vi "ADD ITEM TO CHECKOUT.vi"(10 "REFERENCES":T2, 11 "DATA IN":T1[](array[typedef])) -> (3 "DATA OUT":T1[](array[typedef]))   [LabVIEW 2019]
uses:
  Controls/References Cluster.ctl
  Controls/Custom Calendar/Custom Calendar.xctl
  Controls/Table Data Types/Inventory Data Type.ctl
  <vilib>/addons/database/Connection.llb/DB Tools Open Connec (String).vi
  <vilib>/addons/database/_DB Variant To Data/Database Variant To Data.xnode
  <vilib>/addons/database/NI_Database_API.lvlib
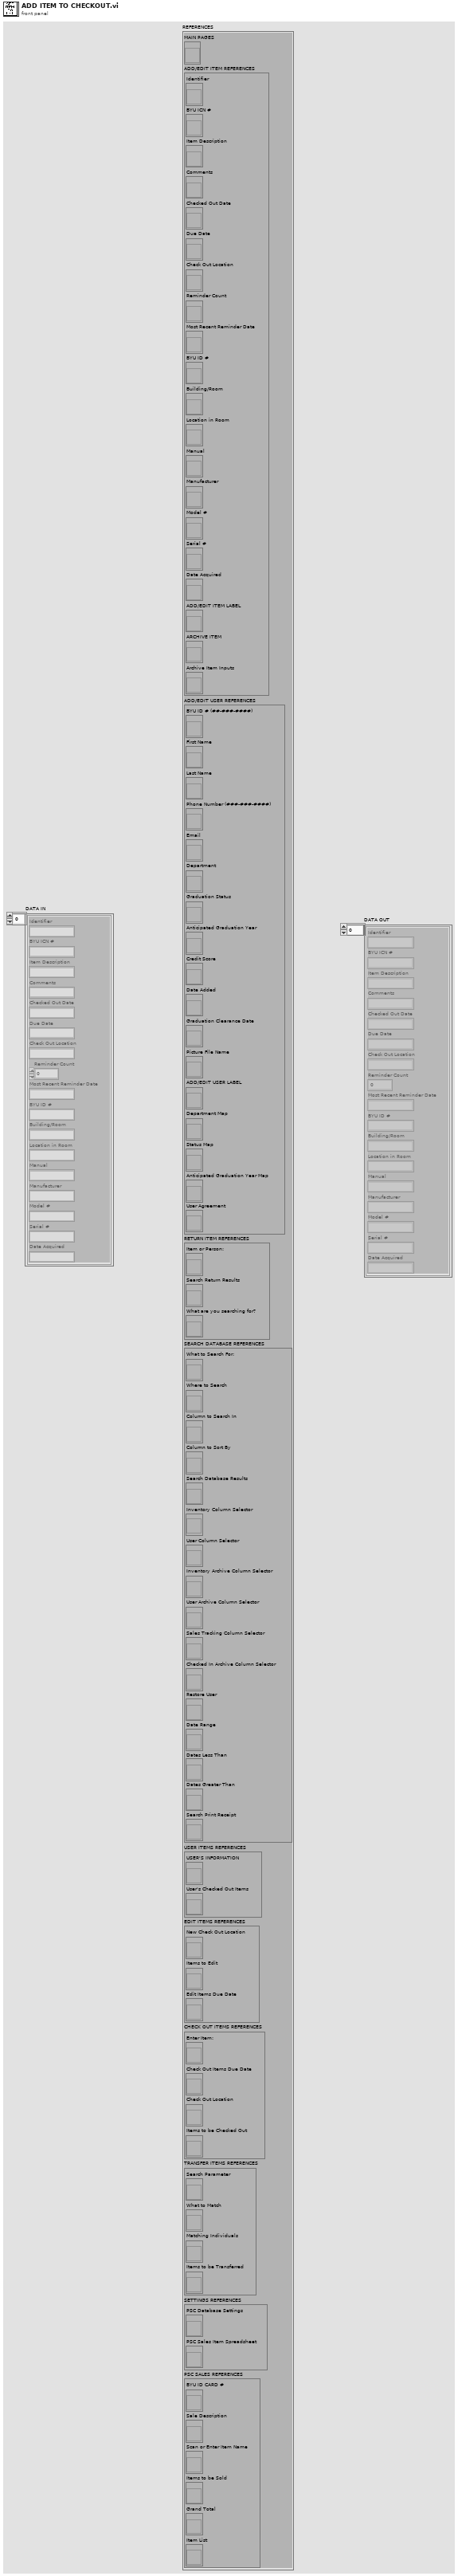
[diagram p1: front panel]
types:
  T1 = typedef "Inventory Data Type.ctl" = cluster{"Identifier":string, "BYU ICN #":string, "Item Description":string, "Comments":string, "Checked Out Date":string, "Due Date":string, "Check Out Location":string, "Reminder Count":i32, "Most Recent Reminder Date":string, "BYU ID #":string, "Building/Room":string, "Location in Room":string, "Manual":string, "Manufacturer":string, "Model #":string, "Serial #":string, "Date Acquired":string}
  T2 = typedef "References Cluster.ctl" = cluster{"MAIN PAGES":refnum<vi>, "ADD/EDIT ITEM REFERENCES":cluster{"Identifier":refnum<vi>, "BYU ICN #":refnum<vi>, "Item Description":refnum<vi>, "Comments":refnum<vi>, "Checked Out Date":refnum<vi>, "Due Date":refnum<vi>, "Check Out Location":refnum<vi>, "Reminder Count":refnum<vi>, "Most Recent Reminder Date":refnum<vi>, "BYU ID #":refnum<vi>, "Building/Room":refnum<vi>, "Location in Room":refnum<vi>, "Manual":refnum<vi>, "Manufacturer":refnum<vi>, "Model #":refnum<vi>, "Serial #":refnum<vi>, "Date Acquired":refnum<vi>, "ADD/EDIT ITEM LABEL":refnum<vi>, "ARCHIVE ITEM":refnum<vi>, "Archive Item Inputs":refnum<vi>}, "ADD/EDIT USER REFERENCES":cluster{"BYU ID # (##-###-####)":refnum<vi>, "First Name":refnum<vi>, "Last Name":refnum<vi>, "Phone Number (###-###-####)":refnum<vi>, "Email":refnum<vi>, "Department":refnum<vi>, "Graduation Status":refnum<vi>, "Anticipated Graduation Year":refnum<vi>, "Credit Score":refnum<vi>, "Date Added":refnum<vi>, "Graduation Clearance Date":refnum<vi>, "Picture File Name":refnum<vi>, "ADD/EDIT USER LABEL":refnum<vi>, "Department Map":refnum<vi>, "Status Map":refnum<vi>, "Anticipated Graduation Year Map":refnum<vi>, "User Agreement":refnum<vi>}, "RETURN ITEM REFERENCES":cluster{"Item or Person:":refnum<vi>, "Search Return Results":refnum<vi>, "What are you searching for?":refnum<vi>}, "SEARCH DATABASE REFERENCES":cluster{"What to Search For:":refnum<vi>, "Where to Search":refnum<vi>, "Column to Search In":refnum<vi>, "Column to Sort By":refnum<vi>, "Search Database Results":refnum<vi>, "Inventory Column Selector":refnum<vi>, "User Column Selector":refnum<vi>, "Inventory Archive Column Selector":refnum<vi>, "User Archive Column Selector":refnum<vi>, "Sales Tracking Column Selector":refnum<vi>, "Checked In Archive Column Selector":refnum<vi>, "Restore User":refnum<vi>, "Date Range":refnum<vi>, "Dates Less Than":refnum<vi>, "Dates Greater Than":refnum<vi>, "Search Print Receipt":refnum<vi>}, "USER ITEMS REFERENCES":cluster{"USER'S INFORMATION":refnum<vi>, "User's Checked Out Items":refnum<vi>}, "EDIT ITEMS REFERENCES":cluster{"New Check Out Location":refnum<vi>, "Items to Edit":refnum<vi>, "Edit Items Due Date":refnum<vi>}, "CHECK OUT ITEMS REFERENCES":cluster{"Enter Item:":refnum<vi>, "Check Out Items Due Date":refnum<vi>, "Check Out Location":refnum<vi>, "Items to be Checked Out":refnum<vi>}, "TRANSFER ITEMS REFERENCES":cluster{"Search Parameter":refnum<vi>, "What to Match":refnum<vi>, "Matching Individuals":refnum<vi>, "Items to be Transferred":refnum<vi>}, "SETTINGS REFERENCES":cluster{"PSC Database Settings":refnum<vi>, "PSC Sales Item Spreadsheet":refnum<vi>}, "PSC SALES REFERENCES":cluster{"BYU ID CARD #":refnum<vi>, "Sale Description":refnum<vi>, "Scan or Enter Item Name":refnum<vi>, "Items to be Sold":refnum<vi>, "Grand Total":refnum<vi>, "Item List":refnum<vi>}}
  T3 = cluster{"Enter Item:":refnum<vi>, "Check Out Items Due Date":refnum<vi>, "Check Out Location":refnum<vi>, "Items to be Checked Out":refnum<vi>}
  T4 = typedef "NI_Database_API.lvlib/Conn ObjectReference.ctl" = refnum<k1>
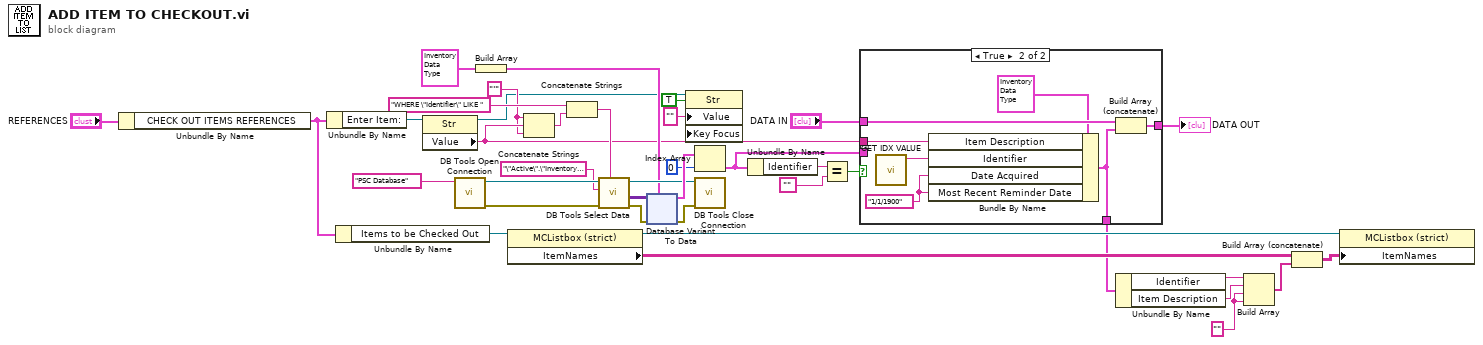
[diagram p0: block diagram]
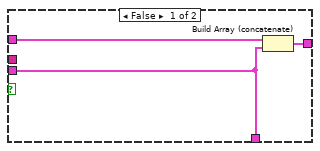
[diagram p2: hidden frame]
diagram:
  w4 = "" ("element")
  w16 = "'"
  n1 = Unbundle By Name("REFERENCES") -> ("CHECK OUT ITEMS REFERENCES"=w14:T3)
  n2 = Unbundle By Name(w14) -> ("Enter Item:"=w37:refnum<vi>)
  n3 = Unbundle By Name(w14) -> ("Items to be Checked Out"=w13:refnum<vi>)
  n4 = property class="Str"(reference=w37) -> (reference out=w3:refnum<vi>, "Value"=w17:string)  [unwired: 1 in, 1 out]
  n5 = call-poly <vilib>:"DB Tools Open Connection.vi"("connection information"="PSC Database") -> ("error out"=w35:errorcluster, "connection reference"=w36:T4)  [unwired: 7 in]
  n6 = Build Array(T1 {"Identifier"="", "BYU ICN #"="", "Item Description"="", "Comments"="", "Checked Out Date"="", "Due Date"="", "Check Out Location"="", "Reminder Count"=0, "Most Recent Reminder Date"="", "BYU ID #"="", "Building/Room"="", "Location in Room"="", "Manual"="", "Manufacturer"="", "Model #"="", "Serial #"="", "Date Acquired"=""} ("Array")) -> (w19:T1[])
  n7 = property class="MCListbox (strict)"(reference=w13) -> (reference out=w8:refnum<vi>, "ItemNames"=w10:string[][])  [unwired: 1 in, 1 out]
  n8 = Concatenate Strings(w16, w17, w16) -> (w18:string)
  n9 = Concatenate Strings("WHERE \"Identifier\" LIKE ", w18) -> (w32:string)
  n10 = call <vilib>:"DB Tools Select Data.vi"("condition"=w32, "error in (no error)"=w35, "table"="\"Active\".\"Inventory\"", "connection reference"=w36) -> ("error out"=w30:errorcluster, "data"=w31:variant[][], "connection reference out"=w27:T4)  [unwired: 2 in]
  n11 = xnode "Database Variant To Data"("database variant"=w31, "error in (no error)"=w30, "type"=w19) -> ("data"=w29:T1[], "error out"=w26:errorcluster)
  n12 = property class="Str"(reference=w3, "Value"="", "Key Focus"=TRUE) -> ()  [unwired: 1 in, 2 out]
  n13 = Index Array(array=w29, index=0) -> (element=w15:T1)
  n14 = call <vilib>:"DB Tools Close Connection.vi"("error in (no error)"=w26, "connection reference"=w27) -> ()  [unwired: 5 in, 1 out]
  n15 = Unbundle By Name(w15) -> ("Identifier"=w25:string)
  n16 = Equal?(x=w25, y="") -> (x = y?=w23:bool)
  n17 = case shown="True" w23 {
    tunnel: "DATA IN" -> [w41 w47]
    tunnel: w15 -> [w39 _]
    tunnel: w17 -> [_ w48]
    tunnel: [w40 w46] -> w21
    tunnel: [w39 w43] -> w6
    frame False {
      n18 = Build Array (concatenate)(w41, w39) -> (w40:T1[])
    }
    frame True {
      w42 = "1/1/1900" ("Date Acquired")
      n19 = call "GET IDX VALUE.vi"() -> ("Identifier Out"=w45:string)  [unwired: 11 in]
      n20 = Bundle By Name(cluster=T1 {"Identifier"="", "BYU ICN #"="", "Item Description"="", "Comments"="", "Checked Out Date"="", "Due Date"="", "Check Out Location"="", "Reminder Count"=0, "Most Recent Reminder Date"="", "BYU ID #"="", "Building/Room"="", "Location in Room"="", "Manual"="", "Manufacturer"="", "Model #"="", "Serial #"="", "Date Acquired"=""} ("INVENTORY DATA TYPE"), "Item Description"=w48, "Identifier"=w45, "Date Acquired"=w42, "Most Recent Reminder Date"=w42) -> (w43:T1)
      n21 = Build Array (concatenate)(w47, w43) -> (w46:T1[])
    }
  }
  "DATA OUT" <- w21
  n22 = Unbundle By Name(w6) -> ("Identifier"=w12:string, "Item Description"=w11:string)
  n23 = Build Array(w12, w11, w4, w4) -> (w9:string[])
  n24 = Build Array (concatenate)(w10, w9) -> (w7:string[][])
  n25 = property class="MCListbox (strict)"(reference=w8, "ItemNames"=w7) -> ()  [unwired: 1 in, 2 out]
